vi "Write Strings to File.vi"(8 "Error In":errorcluster, 9 "Section Name":string, 10 "Array of Strings":string[](array[string]), 11 "Path":path) -> (0 "Error Out":errorcluster)   [LabVIEW 2015]
doc: "This VI was created for use with the Read/Write Cluster VIs. It writes the cluster element strings to the specified section in an INI file without editing any other sections.\n\nFreeware from Moore Good Ideas, www.mooregoodideas.com. Do not remove this line."
uses:
  Suppress Error Code - Scalar.vi
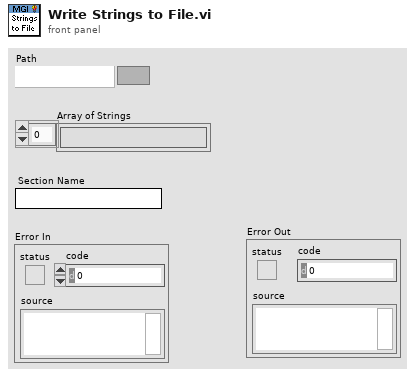
[diagram p1: front panel]
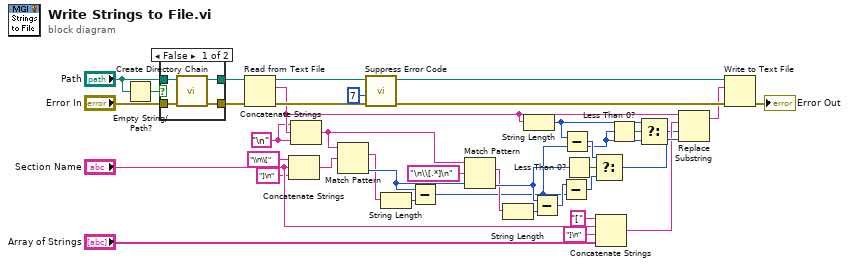
[diagram p0: block diagram]
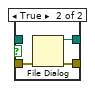
[diagram p2: hidden frame]
diagram:
  w1 = "\n"
  n1 = Empty String/Path?(string/path="Path") -> (empty?=w2:bool)
  n2 = case shown="False" w2 {
    tunnel: "Error In" -> [w41 w44]
    tunnel: [w40 w43] -> w13
    tunnel: [w39 w42] -> w12
    tunnel: "Path" -> [w38 _]
    frame False {
      n3 = call "Create Directory Chain.vi"("Error In"=w41, "Path"=w38) -> ("Error Out"=w40:errorcluster, "Duplicate Path"=w39:path)  [unwired: 8 out]
    }
    frame True {
      n4 = File Dialog(8:w44) -> (0:w43:errorcluster, 3:w42:path)  [unwired: 8 out]
    }
  }
  n5 = Read from Text File(file (use dialog)=w12, error in=w13) -> (text=w11:string, error out=w19:errorcluster)  [unwired: 4 out]
  n6 = Concatenate Strings("\\n\\[" ("string"), "Section Name", "]\n" ("string")) -> (w32:string)
  n7 = Concatenate Strings(w1, w11, w1) -> (w4:string)
  n8 = Match Pattern(string=w4, regular expression=w32) -> (match substring=w22:string, offset past match=w26:i32)  [unwired: 3 out]
  n9 = call-poly "Suppress Error Code.vi"("Error In"=w19, "Error Code"=7) -> ("Error Out"=w36:errorcluster)  [unwired: 9 out]
  n10 = String Length(string=w22) -> (length=w21:i32)
  n11 = Subtract(x=w26, y=w21) -> (x-y=w5:i32)
  n12 = Match Pattern(string=w4, regular expression="\n\\[.*]\n", offset (0)=w26) -> (match substring=w24:string, offset past match=w29:i32)  [unwired: 2 out]
  n13 = String Length(string=w24) -> (length=w23:i32)
  n14 = String Length(string=w11) -> (length=w8:i32)
  n15 = Subtract(x=w29, y=w23) -> (x-y=w25:i32)
  n16 = Subtract(x=w25, y=w5) -> (x-y=w30:i32)
  n17 = Subtract(x=w8, y=w5) -> (x-y=w31:i32)
  n18 = Less Than 0?(x=w29) -> (x < 0?=w28:bool)
  n19 = Select(t=w31, s=w28, f=w30) -> (s? t:f=w27:i32)
  n20 = Concatenate Strings("[" ("string"), "Section Name", "]\n" ("string"), "Array of Strings") -> (w9:string)
  n21 = Less Than 0?(x=w5) -> (x < 0?=w6:bool)
  n22 = Select(t=w8, s=w6, f=w5) -> (s? t:f=w7:i32)
  n23 = Replace Substring(2:w27, 3:w7, 4:w9, 5:w11) -> (1:w10:string)  [unwired: 1 out]
  n24 = Write to Text File(file (use dialog)=w12, text=w10, error in=w36) -> (error out=→"Error Out":errorcluster)  [unwired: 3 out]
